vi "initialaize.vi"(8 "error in (no error)":errorcluster, 9 "Visa com port":refnum<visa-resource-name>, 10 "Serial Device Brand":T1, 11 "Serial Device in":refnum<class "Serial Device.lvclass">) -> (0 "error out":errorcluster, 3 "Serial Device out":refnum<class "Serial Device.lvclass">)   [LabVIEW 2020, in "Serial Device.lvclass"]
uses:
  Serial Device.lvclass
  implementations/Combo box/serial device brand.ctl
  <vilib>/Instr/_visa.llb/VISA Configure Serial Port (Instr).vi
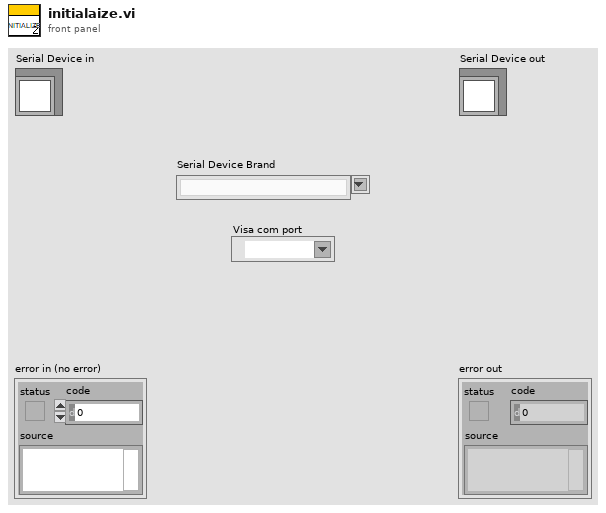
[diagram p1: front panel]
types:
  T1 = typedef "Serial Device.lvclass/serial device brand.ctl" = string
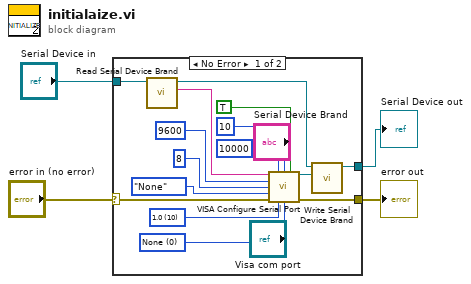
[diagram p0: block diagram]
diagram:
  n1 = case shown="No Error" "error in (no error)" {
    selector: "error in (no error)" -> [w6 w21]
    tunnel: [w5 w21] -> w3
    tunnel: [w17 w20] -> w1
    tunnel: "Serial Device in" -> [w19 w20]
    frame No Error {
      w9 = u16 0 items=["None", "XON/XOFF", "RTS/CTS", "XON/XOFF & RTS/CTS", "DTR/DSR", "XON/XOFF & DTR/DSR"] ("flow control (0:none)")
      w10 = u16 10 items=["1.0"=10, "1.5"=15, "2.0"=20] ("stop bits (10: 1 bit)")
      n2 = call-dynamic "Read Serial Device Brand.vi"("Serial Device in"=w19) -> ("Serial Device Brand"=w7:T1, "Serial Device out"=w18:refnum<class "Serial Device.lvclass">)  [unwired: 8 in, 1 out]
      n3 = call-poly "VISA Configure Serial Port"("VISA resource name"=w7, "timeout (10sec)"=u32 10000, "termination char\n(0xA = '\\n' = LF)"=u8 10 ("termination char\n(0xA = '\\n' = LF)"), "Enable Termination\nChar (T)"=TRUE ("Enable Termination\nChar (T)"), "baud rate (9600)"=u32 9600, "data bits (8)"=u16 8, "parity (0:none)"=enum16{"None", "Odd", "Even", "Mark", "Space"}."None", "error in (no error)"=w6, "stop bits (10: 1 bit)"=w10, "flow control (0:none)"=w9) -> ("VISA resource name out"=w8:refnum<visa-resource-name>, "error out"=w5:errorcluster)  [unwired: 4 in]
      n4 = call-dynamic "Write Serial Device Brand.vi"("Serial Device Brand"=w8, "Serial Device in"=w18) -> ("Serial Device out"=w17:refnum<class "Serial Device.lvclass">)  [unwired: 8 in, 1 out]
    }
    frame Error {
    }
  }
  "error out" <- w3
  "Serial Device out" <- w1
